vi "GetVIText.vi"(8 "error in (no error)":errorcluster, 10 "Control Name (Blank = All controls in VI)":string, 11 "VI":refnum<vi>) -> (0 "error out":errorcluster, 2 "Control UIDs":string[](array[string]), 3 "Control Text":string[](array[string]))   [LabVIEW 2017]
uses:
  <vilib>/Utility/traverseref.llb/TRef TravTarget.ctl
  <vilib>/Utility/traverseref.llb/VI Scripting - Traverse.lvlib
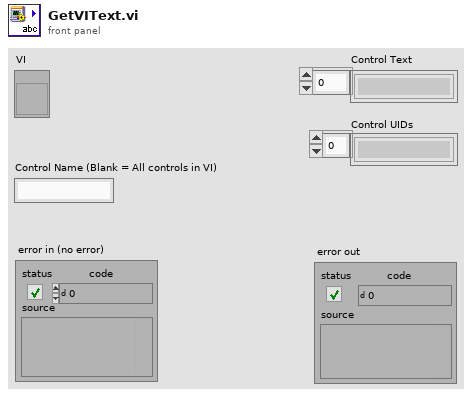
[diagram p1: front panel]
types:
  T1 = typedef "TRef TravTarget.ctl" = enum16{"FP", "BD", "Other"}
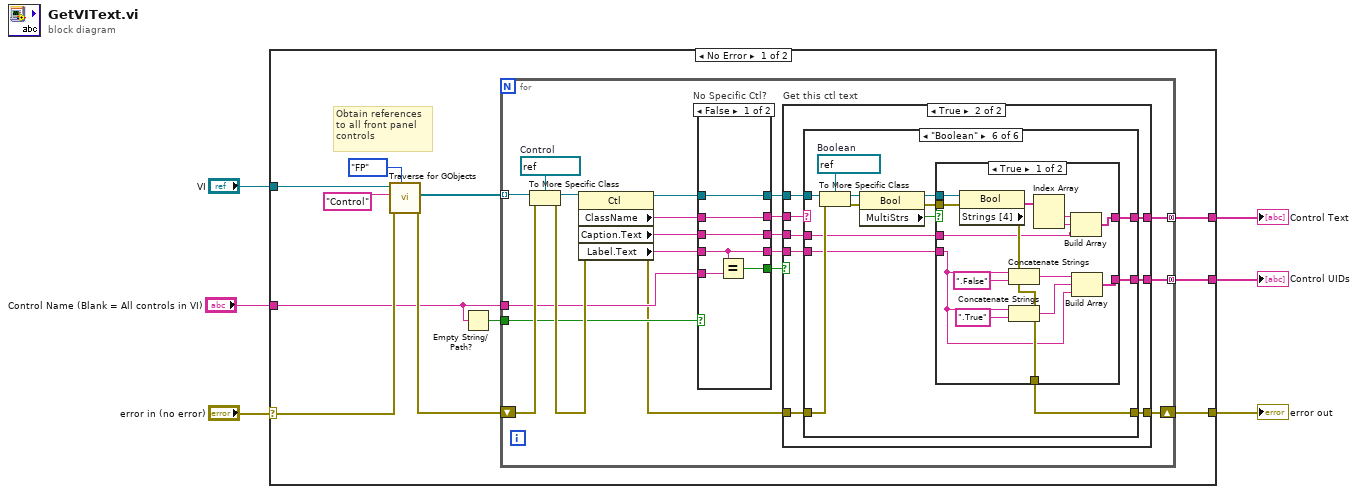
[diagram p0: block diagram]
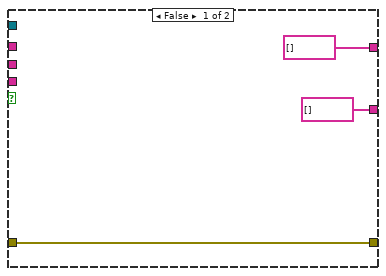
[diagram p2: hidden frame]
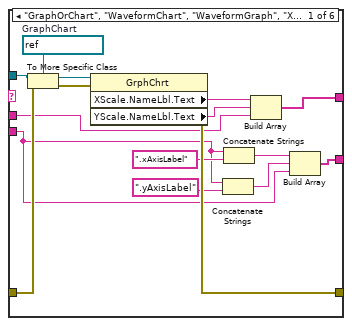
[diagram p3: hidden frame]
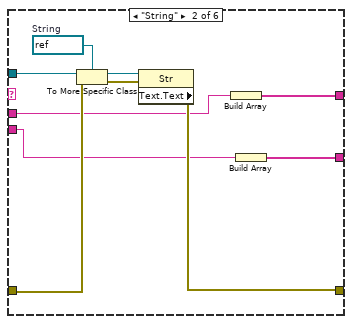
[diagram p4: hidden frame]
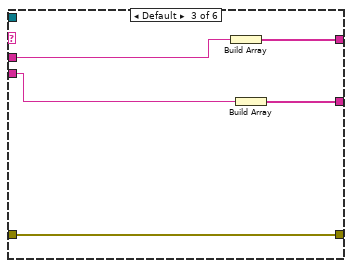
[diagram p5: hidden frame]
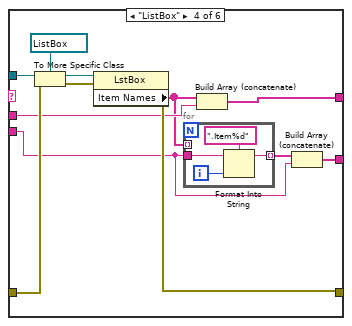
[diagram p6: hidden frame]
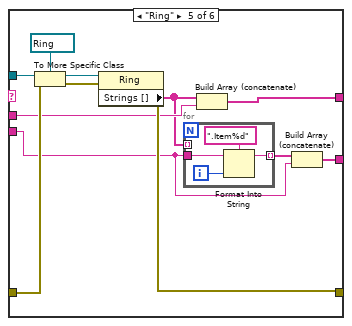
[diagram p7: hidden frame]
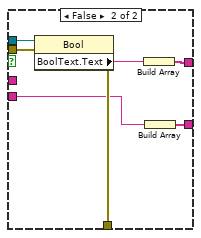
[diagram p8: hidden frame]
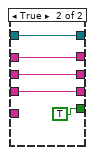
[diagram p9: hidden frame]
diagram:
  n1 = case shown="No Error" "error in (no error)" {
    selector: "error in (no error)" -> [w13 w157]
    tunnel: "VI" -> [w15 _]
    tunnel: "Control Name (Blank = All controls in VI)" -> [w9 _]
    tunnel: [w11 w157] -> w3
    tunnel: [w8 _] -> w2
    tunnel: [w7 _] -> w1
    frame No Error {
      # "Obtain references to all front panel controls"
      n2 = call <vilib>:"Traverse for GObjects.vi"("Traverse Target"=TRef_TravTarget."FP", "error in (no error)"=w13, "Class Name"="Control", "VI Refnum"=w15) -> ("error out"=w12:errorcluster, "References"=w14:refnum<vi>[])  [unwired: 4 in, 2 out]
      n3 = Empty String/Path?(string/path=w9) -> (empty?=w10:bool)
      n4 = for {
        tunnel: w14 -> [w37] mode=indexing
        shift-right: [w26] -> w11
        shift-left: w12 -> [w34]
        tunnel: w9 -> [w32]
        tunnel: w10 -> [w30]
        tunnel: [w19] -> w8 mode=concatenating
        tunnel: [w18] -> w7 mode=concatenating
        w35 = refnum<vi> refnum  # Control
        n5 = To More Specific Class(target class=w35, reference=w37, error in=w34) -> (specific class reference=w36:refnum<vi>, error out=w33:errorcluster)
        n6 = property class="Ctl"(reference=w36, error in=w33) -> (reference out=w20:refnum<vi>, error out=w27:errorcluster, "ClassName"=w29:string, "Caption.Text"=w28:string, "Label.Text"=w31:string)
        n7 = case "No Specific Ctl?" shown="False" w30 {
          tunnel: w32 -> [w151 _]
          tunnel: w31 -> [w149 w153]
          tunnel: w29 -> [w147 w156]
          tunnel: w28 -> [w148 w154]
          tunnel: [w150 TRUE] -> w25
          tunnel: [w147 w156] -> w22
          tunnel: [w148 w154] -> w24
          tunnel: [w149 w153] -> w23
          tunnel: [w146 w152] -> w21
          tunnel: w20 -> [w146 w152]
          frame False {
            n8 = Equal?(x=w149, y=w151) -> (x = y?=w150:bool)
          }
          frame True {
          }
        }
        n9 = case "Get this ctl text" shown="True" w25 {
          tunnel: w27 -> [w40 w46]
          tunnel: [w40 w45] -> w26
          tunnel: w24 -> [_ w43]
          tunnel: w23 -> [_ w44]
          tunnel: w22 -> [_ w48]
          tunnel: w21 -> [_ w47]
          tunnel: [string[] [] w42] -> w19
          tunnel: [string[] [] w41] -> w18
          frame False {
          }
          frame True {
            n10 = case shown="\"Boolean\"" w48 {
              tunnel: w47 -> [w61 w71 _ w88 w104 w123]
              tunnel: w46 -> [w60 w70 w79 w87 w103 w122]
              tunnel: [w59 w69 w79 w86 w102 w121] -> w45
              tunnel: [w58 w68 w78 w85 w101 w120] -> w42
              tunnel: w44 -> [w50 w66 w76 w81 w97 w118]
              tunnel: w43 -> [w57 w67 w77 w84 w100 w119]
              tunnel: [w49 w65 w75 w80 w96 w117] -> w41
              frame "GraphOrChart", "WaveformChart", "WaveformGraph", "XYGraph" {
                w63 = refnum<vi> refnum  # GraphChart
                n11 = To More Specific Class(target class=w63, reference=w61, error in=w60) -> (specific class reference=w64:refnum<vi>, error out=w62:errorcluster)
                n12 = property class="GrphChrt"(reference=w64, error in=w62) -> (error out=w59:errorcluster, "XScale.NameLbl.Text"=w54:string, "YScale.NameLbl.Text"=w53:string)  [unwired: 1 out]
                n13 = Concatenate Strings(w50, ".yAxisLabel" ("string")) -> (w51:string)
                n14 = Concatenate Strings(w50, ".xAxisLabel" ("string")) -> (w52:string)
                n15 = Build Array(w54, w53, w57) -> (w58:string[])
                n16 = Build Array(w52, w51, w50) -> (w49:string[])
              }
              frame "String" {
                w74 = refnum<vi> refnum  # String
                n17 = To More Specific Class(target class=w74, reference=w71, error in=w70) -> (specific class reference=w73:refnum<vi>, error out=w72:errorcluster)
                n18 = property class="Str" props=["Text", "Text"](reference=w73, error in=w72) -> (error out=w69:errorcluster)  [unwired: 2 out]
                n19 = Build Array(w67) -> (w68:string[])
                n20 = Build Array(w66) -> (w65:string[])
              }
              frame Default {
                n21 = Build Array(w77) -> (w78:string[])
                n22 = Build Array(w76) -> (w75:string[])
              }
              frame "ListBox" {
                n23 = To More Specific Class(target class=refnum<vi> refnum ("reference out"), reference=w88, error in=w87) -> (specific class reference=w91:refnum<vi>, error out=w90:errorcluster)
                n24 = property class="LstBox"(reference=w91, error in=w90) -> (error out=w86:errorcluster, "Item Names"=w83:string[])  [unwired: 1 out]
                n25 = for {
                  tunnel: w81 -> [w95]
                  tunnel: w83 -> [_] mode=indexing
                  tunnel: [w92] -> w82 mode=indexing
                  i -> [w93]
                  n26 = Format Into String(format string=".Item%d", initial string=w95, w93) -> (resulting string=w92:string)  [unwired: 1 in, 1 out]
                }
                n27 = Build Array (concatenate)(w83, w84) -> (w85:string[])
                n28 = Build Array (concatenate)(w82, w81) -> (w80:string[])
              }
              frame "Ring" {
                n29 = To More Specific Class(target class=refnum<vi> refnum ("reference out"), reference=w104, error in=w103) -> (specific class reference=w107:refnum<vi>, error out=w106:errorcluster)
                n30 = property class="Ring"(reference=w107, error in=w106) -> (error out=w102:errorcluster, "Strings []"=w99:string[])  [unwired: 1 out]
                n31 = for {
                  tunnel: w97 -> [w111]
                  tunnel: w99 -> [_] mode=indexing
                  tunnel: [w108] -> w98 mode=indexing
                  i -> [w109]
                  n32 = Format Into String(format string=".Item%d", initial string=w111, w109) -> (resulting string=w108:string)  [unwired: 1 in, 1 out]
                }
                n33 = Build Array (concatenate)(w99, w100) -> (w101:string[])
                n34 = Build Array (concatenate)(w98, w97) -> (w96:string[])
              }
              frame "Boolean" {
                w124 = refnum<vi> refnum  # Boolean
                n35 = To More Specific Class(target class=w124, reference=w123, error in=w122) -> (specific class reference=w116:refnum<vi>, error out=w114:errorcluster)
                n36 = property class="Bool"(reference=w116, error in=w114) -> (reference out=w115:refnum<vi>, error out=w113:errorcluster, "MultiStrs"=w112:bool)
                n37 = case shown="True" w112 {
                  tunnel: [w138 w140] -> w121
                  tunnel: [w136 w144] -> w120
                  tunnel: w119 -> [w125 _]
                  tunnel: w118 -> [w131 w139]
                  tunnel: [w130 w143] -> w117
                  tunnel: w115 -> [w129 w142]
                  tunnel: w113 -> [w128 w141]
                  frame True {
                    n38 = property class="Bool"(reference=w129, error in=w128) -> (error out=w138:errorcluster, "Strings [4]"=w137:string[])  [unwired: 1 out]
                    n39 = Concatenate Strings(w131, ".False" ("string")) -> (w134:string)
                    n40 = Concatenate Strings(w131, ".True" ("string")) -> (w132:string)
                    n41 = Index Array(array=w137) -> (element #1=w127:string, element #2=w126:string)  [unwired: 2 in]
                    n42 = Build Array(w127, w126, w125) -> (w136:string[])
                    n43 = Build Array(w134, w132, w131) -> (w130:string[])
                  }
                  frame False {
                    n44 = property class="Bool"(reference=w142, error in=w141) -> (error out=w140:errorcluster, "BoolText.Text"=w145:string)  [unwired: 1 out]
                    n45 = Build Array(w145) -> (w144:string[])
                    n46 = Build Array(w139) -> (w143:string[])
                  }
                }
              }
            }
          }
        }
      }
    }
    frame Error {
    }
  }
  "Control Text" <- w2
  "error out" <- w3
  "Control UIDs" <- w1
